vi "KP_KI_Integration.vi"() -> ()   [LabVIEW 2023]
panel:
  out "Ki":dbl
  out "Kp":dbl
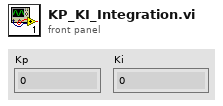
[diagram p1: front panel]
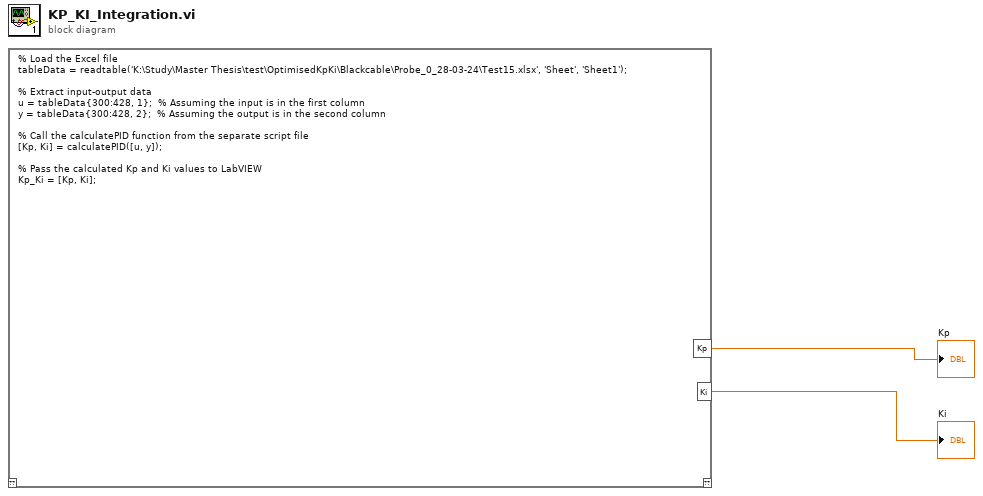
[diagram p0: block diagram]
diagram:
  n1 = script code="% Load the Excel file\ntableData = readtable('K:\\Study\\Master Thesis\\test\\OptimisedKpKi\\Blackcable\\Probe_0_28-03-24\\Test15.xlsx', 'Sheet', 'Sheet1');\n\n% Extract input-output data\nu = tableData{300:428, 1};  % Assuming the input is in the first column\ny = tableData{300:428, 2};  % Assuming the output is in the second column\n\n% Call the calculatePID function from the separate script file\n[Kp, Ki] = calculatePID([u, y]);\n\n% Pass the calculated Kp and Ki values to LabVIEW\nKp_Ki = [Kp, Ki];"() -> ("Kp"=→"Kp":dbl, "Ki"=→"Ki":dbl)  [unwired: 1 in, 1 out]
